vi "Rectangle Size.vi"(11 "Rectangle":T1) -> (1 "Point?":bool, 2 "Line?":bool, 3 "Rect Size":cluster{"width":i32, "height":i32})   [LabVIEW 2012]
doc: "Calculates the center of a rectangle"
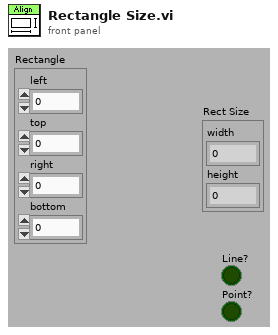
[diagram p1: front panel]
types:
  T1 = cluster{"left":i16, "top":i16, "right":i16, "bottom":i16}
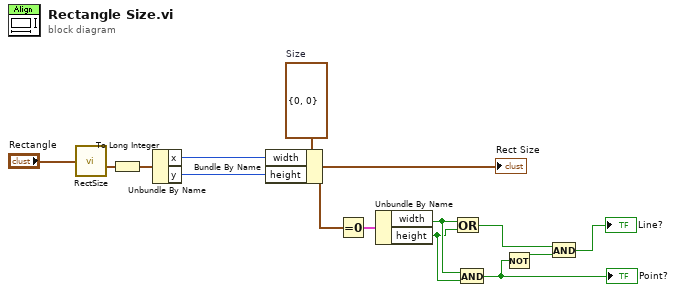
[diagram p0: block diagram]
diagram:
  w14 = cluster{"width":i32, "height":i32} {"width"=0, "height"=0}  # Size
  n1 = call <vilib>:"RectSize.vi"("rect"="Rectangle") -> ("point"=w12:cluster{"x":i16, "y":i16})
  n2 = To Long Integer(number=w12) -> (32bit integer=w11:cluster{"x":i32, "y":i32})
  n3 = Unbundle By Name(w11) -> ("x"=w10:i32, "y"=w9:i32)
  n4 = Bundle By Name(cluster=w14, "width"=w10, "height"=w9) -> (w8:cluster{"width":i32, "height":i32})
  "Rect Size" <- w8
  n5 = Equal To 0?(x=w8) -> (x = 0?=w7:cluster{"width":bool, "height":bool})
  n6 = Unbundle By Name(w7) -> ("width"=w6:bool, "height"=w5:bool)
  n7 = Or(x=w6, y=w5) -> (x .or. y?=w2:bool)
  n8 = And(x=w6, y=w5) -> (x .and. y?=w3:bool)
  "Point?" <- w3
  n9 = Not(x=w3) -> (.not. x?=w4:bool)
  n10 = And(x=w2, y=w4) -> (x .and. y?=→"Line?":bool)
